vi "功能试验 扭矩变化峰值.vi"(9 "扭矩正转2":dbl[](array[numeric]), 10 "扭矩反转":dbl[](array[numeric]), 11 "扭矩正转":dbl[](array[numeric])) -> (2 "反转扭矩变化峰值":dbl, 3 "正转扭矩变化峰值":dbl)   [LabVIEW 2015, in "Logging.lvlib"]
uses:
  Logging.lvlib
  <vilib>/Analysis/NI_AAL_SigProc.lvlib
  <vilib>/Analysis/NI_AALBase.lvlib
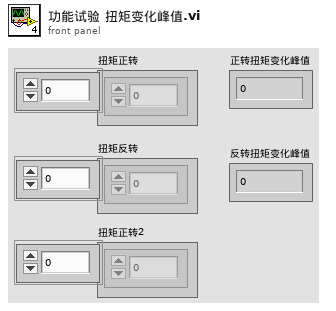
[diagram p1: front panel]
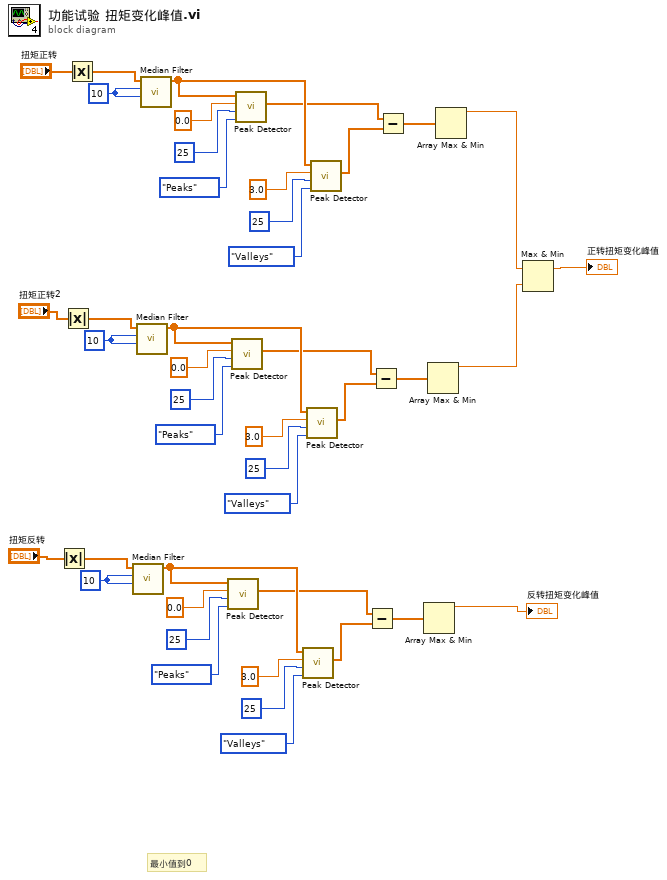
[diagram p0: block diagram]
diagram:
  w22 = 10 ("left rank")
  w34 = 10 ("left rank")
  w43 = 10 ("left rank")
  # "最小值到0"
  n1 = Absolute Value(x="扭矩反转") -> (abs(x)=w15:dbl[])
  n2 = Absolute Value(x="扭矩正转2") -> (abs(x)=w24:dbl[])
  n3 = Absolute Value(x="扭矩正转") -> (abs(x)=w8:dbl[])
  n4 = call <vilib>:"Median Filter.vi"("right rank"=w22, "left rank"=w22, "X"=w15) -> ("Filtered X"=w14:dbl[])  [unwired: 7 in, 1 out]
  n5 = call <vilib>:"Median Filter.vi"("right rank"=w34, "left rank"=w34, "X"=w24) -> ("Filtered X"=w7:dbl[])  [unwired: 7 in, 1 out]
  n6 = call <vilib>:"Median Filter.vi"("right rank"=w43, "left rank"=w43, "X"=w8) -> ("Filtered X"=w9:dbl[])  [unwired: 7 in, 1 out]
  n7 = call <vilib>:"Peak Detector.vi"("peaks/valleys"=enum32{"Peaks", "Valleys"}."Peaks", "width"=25, "threshold"=0.0, "X"=w14) -> ("Amplitudes"=w2:dbl[])  [unwired: 3 in, 4 out]
  n8 = call <vilib>:"Peak Detector.vi"("peaks/valleys"=enum32{"Peaks", "Valleys"}."Peaks", "width"=25, "threshold"=0.0, "X"=w7) -> ("Amplitudes"=w4:dbl[])  [unwired: 3 in, 4 out]
  n9 = call <vilib>:"Peak Detector.vi"("peaks/valleys"=enum32{"Peaks", "Valleys"}."Peaks", "width"=25, "threshold"=0.0, "X"=w9) -> ("Amplitudes"=w6:dbl[])  [unwired: 3 in, 4 out]
  n10 = call <vilib>:"Peak Detector.vi"("peaks/valleys"=enum32{"Peaks", "Valleys"}."Valleys", "width"=25, "threshold"=3.0, "X"=w14) -> ("Amplitudes"=w1:dbl[])  [unwired: 3 in, 4 out]
  n11 = call <vilib>:"Peak Detector.vi"("peaks/valleys"=enum32{"Peaks", "Valleys"}."Valleys", "width"=25, "threshold"=3.0, "X"=w7) -> ("Amplitudes"=w3:dbl[])  [unwired: 3 in, 4 out]
  n12 = call <vilib>:"Peak Detector.vi"("peaks/valleys"=enum32{"Peaks", "Valleys"}."Valleys", "width"=25, "threshold"=3.0, "X"=w9) -> ("Amplitudes"=w5:dbl[])  [unwired: 3 in, 4 out]
  n13 = Subtract(x=w2, y=w1) -> (x-y=w13:dbl[])
  n14 = Subtract(x=w4, y=w3) -> (x-y=w23:dbl[])
  n15 = Subtract(x=w6, y=w5) -> (x-y=w35:dbl[])
  n16 = Array Max & Min(array=w13) -> (max value=→"反转扭矩变化峰值":dbl)  [unwired: 3 out]
  n17 = Array Max & Min(array=w23) -> (max value=w26:dbl)  [unwired: 3 out]
  n18 = Array Max & Min(array=w35) -> (max value=w27:dbl)  [unwired: 3 out]
  n19 = Max & Min(x=w27, y=w26) -> (max(x,y)=→"正转扭矩变化峰值":dbl)  [unwired: 1 out]
